vi "icListen 4 Enabled.vi"() -> ()   [LabVIEW 2020, in "PAM Library.lvlib"]
uses:
  PAM Library.lvlib
panel:
  in  "icListen 4 Enabled":bool
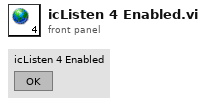
[diagram p1: front panel]
diagram:
